vi "GetPrimaryDisplay.vi"(8 "No Error":errorcluster) -> (0 "Error Out":errorcluster, 3 "DisplayID":T1)   [LabVIEW 2024, in "SDL3.lvlib" / "Video.lvlib"]
doc: "<B>Summary</B>\nReturn the primary display."
uses:
  Video.lvlib
  Lib/SDL3-32.dll
  Error/Error.lvlib
  DisplayID--integer.ctl
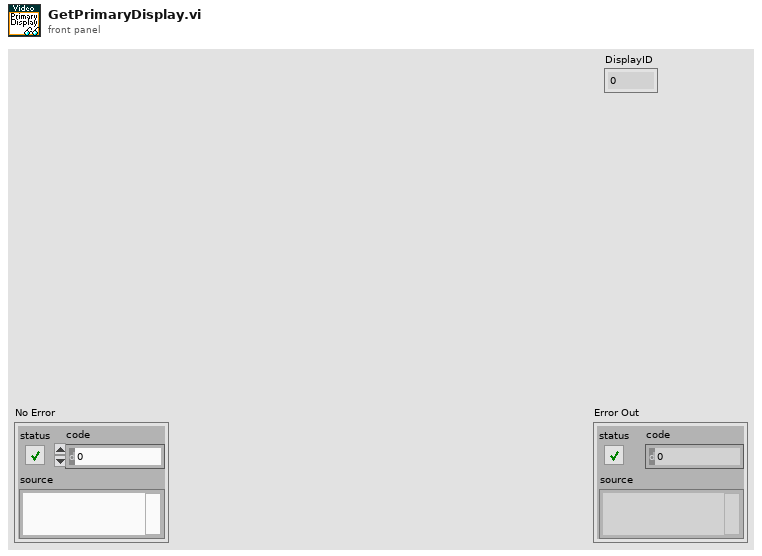
[diagram p1: front panel]
types:
  T1 = typedef "SDL3.lvlib/Video.lvlib/DisplayID--integer.ctl" = u32
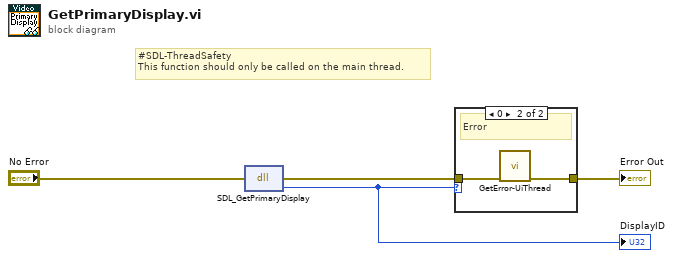
[diagram p0: block diagram]
diagram:
  # "#SDL-ThreadSafety\nThis function should only be called on the main thread."
  n1 = dll-call lib="C:/Users/Thomas/Documents/Projects/LV-SDL3/Lib/SDL3-*.*" fn="SDL_GetPrimaryDisplay"(error in="No Error") -> (error out=w2:errorcluster, "return type"=w1:u32)  [unwired: 2 in, 1 out]
  "DisplayID" <- w1
  n2 = case shown="0" w1 {
    tunnel: w2 -> [w5 w7]
    tunnel: [w5 w6] -> w3
    frame Default {
      # "Ok"
    }
    frame 0 {
      # "Error"
      n3 = call "GetError-UiThread.vi"("No Error"=w7) -> ("error out"=w6:errorcluster)  [unwired: 10 in]
    }
  }
  "Error Out" <- w3
